vi "SysInfo-Get Fixed Drives.vi"(11 "Error In":errorcluster) -> (8 "Fixed drives":string[](array[string]), 15 "error IO":errorcluster)   [LabVIEW 2020]
uses:
  C:/Users/kehan/Downloads/Drive Type.ctl
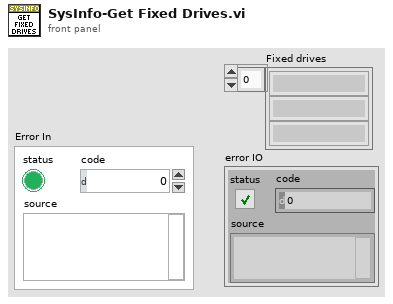
[diagram p1: front panel]
types:
  T1 = typedef "SysInfo-Drive Info.ctl" = cluster{"Drive":string, "DriveType":T2, "VolumeLabel":string, "DriveFormat":string, "IsReady":bool}
  T2 = typedef "Drive Type.ctl" = enum16{"Unknown", "NoRootDirectory", "Removable", "Fixed", "Network", "CDRom", "Ram"}
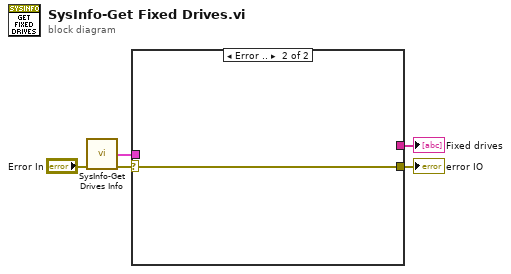
[diagram p0: block diagram]
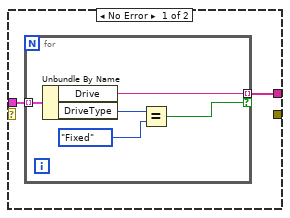
[diagram p2: hidden frame]
diagram:
  n1 = call "SysInfo-Get Drives Info.vi"("Error In"="Error In") -> ("Array"=w5:T1[], "Error Out"=w3:errorcluster)  [unwired: 13 in]
  n2 = case shown="Error .." w3 {
    selector: w3 -> [_ w13]
    tunnel: w5 -> [w7 _]
    tunnel: [w6 _] -> w2
    tunnel: [_ w13] -> w1
    frame No Error {
      n3 = for {
        tunnel: w7 -> [w12] mode=indexing
        tunnel: [w11] -> w6 mode=indexing if=w8
        n4 = Unbundle By Name(w12) -> ("Drive"=w11:string, "DriveType"=w10:T2)
        n5 = Equal?(x=w10, y=Drive_Type."Fixed") -> (x = y?=w8:bool)
      }
    }
    frame Error {
    }
  }
  "Fixed drives" <- w2
  "error IO" <- w1
